vi "FlatToRichnixnet_grpc_FrameRequest.vi"(5 "OutputClusterType":T1, 11 "InputCluster":T3) -> (3 "OutputCluster":T1)   [LabVIEW 2025, in "xnet-grpc_client.lvlib"]
uses:
  nixnet_grpc_FrameRequest_Flat.ctl
  nixnet_grpc_FrameType.ctl
  nixnet_grpc_FrameFlags.ctl
  nixnet_grpc_FrameRequest.ctl
  nixnet_grpc_FrameRequest_type_enum/nixnet_grpc_FrameRequest_type_enum.lvclass
  xnet-grpc_client.lvlib
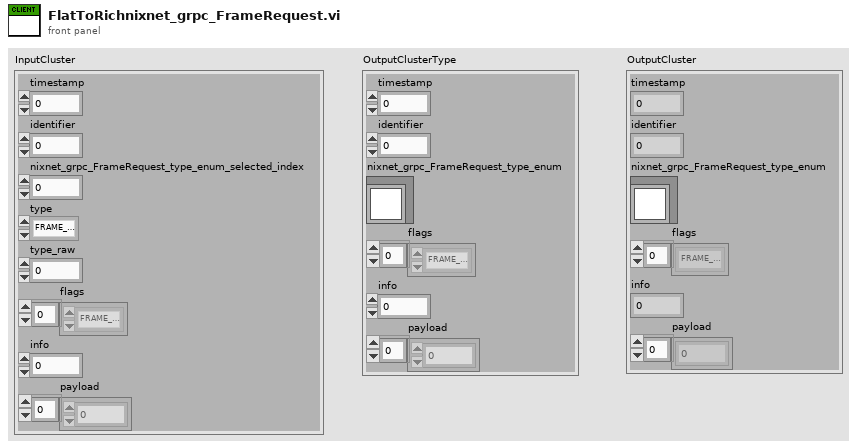
[diagram p1: front panel]
types:
  T1 = typedef "xnet-grpc_client.lvlib/nixnet_grpc_FrameRequest.ctl" = cluster{"timestamp":u64, "identifier":u32, "nixnet_grpc_FrameRequest_type_enum":refnum<class "nixnet_grpc_FrameRequest_type_enum.lvclass">, "flags":T2[], "info":u32, "payload":u8[]}
  T2 = typedef "xnet-grpc_client.lvlib/nixnet_grpc_FrameFlags.ctl" = enum32{"FRAME_FLAGS_UNSPECIFIED", "FRAME_FLAGS_FLEX_RAY_STARTUP", "FRAME_FLAGS_FLEX_RAY_SYNC", "FRAME_FLAGS_FLEX_RAY_PREAMBLE", "FRAME_FLAGS_FLEX_RAY_CH_A", "FRAME_FLAGS_FLEX_RAY_CH_B", "FRAME_FLAGS_LIN_EVENT_SLOT", "FRAME_FLAGS_TRANSMIT_ECHO"}
  T3 = typedef "xnet-grpc_client.lvlib/nixnet_grpc_FrameRequest_Flat.ctl" = cluster{"timestamp":u64, "identifier":u32, "nixnet_grpc_FrameRequest_type_enum_selected_index":i32, "type":T4, "type_raw":u32, "flags":T2[], "info":u32, "payload":u8[]}
  T4 = typedef "xnet-grpc_client.lvlib/nixnet_grpc_FrameType.ctl" = enum32{"FRAME_TYPE_CAN_DATA", "FRAME_TYPE_CAN_REMOTE", "FRAME_TYPE_CAN_BUS_ERROR", "FRAME_TYPE_CAN20_DATA", "FRAME_TYPE_CANFD_DATA", "FRAME_TYPE_CANFDBRS_DATA", "FRAME_TYPE_FLEX_RAY_DATA", "FRAME_TYPE_FLEX_RAY_NULL", "FRAME_TYPE_FLEX_RAY_SYMBOL", "FRAME_TYPE_LIN_DATA", "FRAME_TYPE_LIN_BUS_ERROR", "FRAME_TYPE_LIN_NO_RESPONSE", "FRAME_TYPE_J1939_DATA", "FRAME_TYPE_SPECIAL_DELAY", "FRAME_TYPE_SPECIAL_LOG_TRIGGER", "FRAME_TYPE_SPECIAL_START_TRIGGER"}
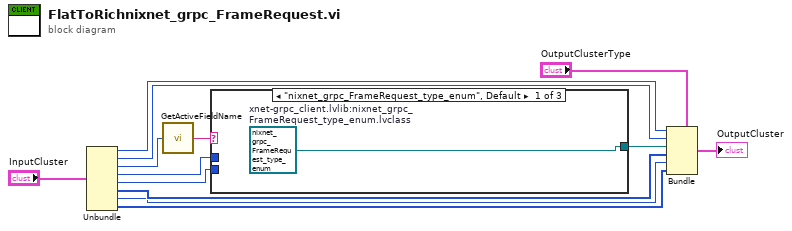
[diagram p0: block diagram]
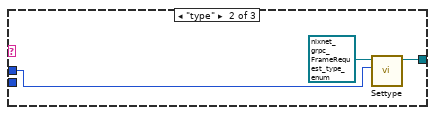
[diagram p2: hidden frame]
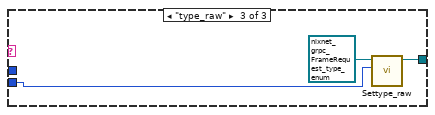
[diagram p3: hidden frame]
diagram:
  n1 = Unbundle "Unbundle"("InputCluster") -> ("timestamp"=w10:u64, "identifier"=w9:u32, "nixnet_grpc_FrameRequest_type_enum_selected_index"=w8:i32, "type"=w5:T4, "type_raw"=w4:u32, "flags"=w3:T2[], "info"=w2:u32, "payload"=w1:u8[])
  n2 = call "GetActiveFieldName.vi"("protobuf index"=w8) -> ("oneof field name"=w7:string)
  n3 = case "nixnet_grpc_FrameRequest_type_enum" shown="\"nixnet_grpc_FrameRequest_type_enum\", Default" w7 {
    tunnel: [w14 w16 w19] -> w6
    tunnel: w5 -> [_ w17 _]
    tunnel: w4 -> [_ _ w20]
    frame "nixnet_grpc_FrameRequest_type_enum", Default {
      w14 = refnum<class "nixnet_grpc_FrameRequest_type_enum.lvclass"> refnum  # xnet-grpc_client.lvlib:nixnet_grpc_FrameRequest_type_enum.lvclass
    }
    frame "type" {
      n4 = call "Settype.vi"("Set_Val"=w17, "OneOfTemplate in"=refnum<class "nixnet_grpc_FrameRequest_type_enum.lvclass"> refnum) -> ("OneOfTemplate out"=w16:refnum<class "nixnet_grpc_FrameRequest_type_enum.lvclass">)  [unwired: 8 in, 1 out]
    }
    frame "type_raw" {
      n5 = call "Settype_raw.vi"("Set_Val"=w20, "OneOfTemplate in"=refnum<class "nixnet_grpc_FrameRequest_type_enum.lvclass"> refnum) -> ("OneOfTemplate out"=w19:refnum<class "nixnet_grpc_FrameRequest_type_enum.lvclass">)  [unwired: 8 in, 1 out]
    }
  }
  n6 = Bundle "Bundle"(cluster="OutputClusterType", "timestamp"=w10, "identifier"=w9, "nixnet_grpc_FrameRequest_type_enum"=w6, "flags"=w3, "info"=w2, "payload"=w1) -> (→"OutputCluster":T1)
